vi "RN_Motorstrom.vi"(6 "error in":errorcluster, 7 "Stromstärke in mA / 10":u8=10 max=200 step=1, 8 "Motorwahl":string(combo)="0", 9 "VISA resource name in":refnum<visa-resource-name>) -> (0 "error out":errorcluster, 2 "Gesendeter Code":string, 3 "VISA resource name out":refnum<visa-resource-name>)   [LabVIEW 2014]
doc: "VI zum Einstellen des Motorstroms der RI-Motorsteuerung;\n\nStromstärke in mA / 10 (Bsp.: für 1900mA muss 190 angegeben werden)\n\nStandardwert: 100mA (=10)"
panel:
  in  "Steuercode":string="i"
  in  "Kennung - RN-Motorsteuerung":string="#rm"
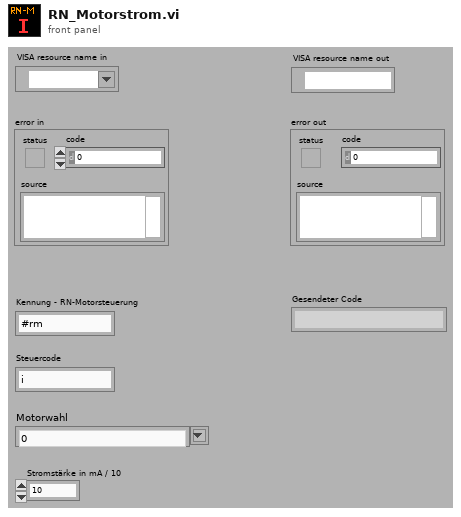
[diagram p1: front panel]
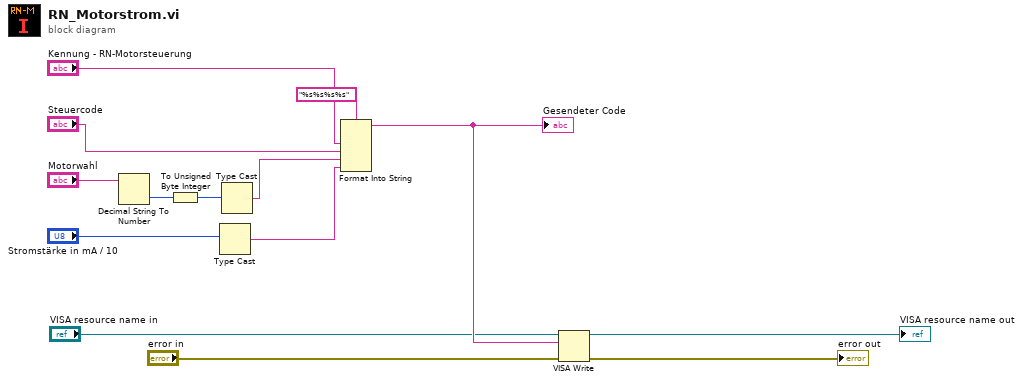
[diagram p0: block diagram]
diagram:
  n1 = Decimal String To Number(string="Motorwahl") -> (number=w13:i32)  [unwired: 2 in, 1 out]
  n2 = To Unsigned Byte Integer(number=w13) -> (unsigned 8bit integer=w12:u8)
  n3 = Type Cast(x="Stromstärke in mA / 10") -> (*(type *) &x=w7:string)  [unwired: 1 in]
  n4 = Type Cast(x=w12) -> (*(type *) &x=w8:string)  [unwired: 1 in]
  n5 = Format Into String(format string="%s%s%s%s", "Kennung - RN-Motorsteuerung", "Steuercode", w8, w7) -> (resulting string=w5:string)  [unwired: 2 in, 1 out]
  "Gesendeter Code" <- w5
  n6 = VISA Write(VISA resource name="VISA resource name in", write buffer=w5, error in (no error)="error in") -> (VISA resource name out=→"VISA resource name out":refnum<visa-resource-name>, error out=→"error out":errorcluster)  [unwired: 1 out]
